vi "Save.vi"(0 "User Manager Model in":refnum<class "User Manager Model.lvclass">, 11 "error in (no error)":errorcluster) -> (4 "User Manager Model out":refnum<class "User Manager Model.lvclass">, 15 "error out":errorcluster)   [LabVIEW 2017, in "User Manager Model.lvlib" / "User Manager Model.lvclass"]
uses:
  User Manager Model.lvclass
  <vilib>/gpm_packages/@cs/persistence/source/XML/XML.lvclass
  C:/Program Files/National Instruments/LabVIEW 2017/vi.lib/gpm_packages/@cs/persistence/source/IPersist/IPersist.lvclass
  User Manager Model.lvclass/User Manager Model.ctl
  Accessors/Read Persistence Path.vi
  <vilib>/gpm_packages/@cs/user-manager/Source/User Configuration Manager Ref/By Ref.lvlib
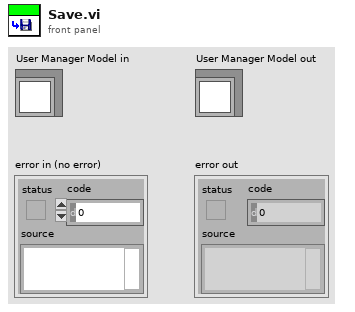
[diagram p1: front panel]
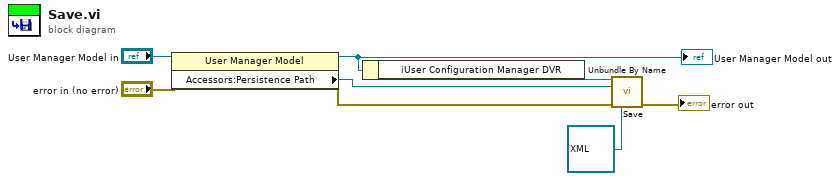
[diagram p0: block diagram]
diagram:
  n1 = property on="Property Node" class="User Manager Model"(reference="User Manager Model in", error in="error in (no error)") -> (reference out=w5:refnum<class "User Manager Model.lvclass">, error out=w2:errorcluster, "Accessors:Persistence Path"=w3:path)
  "User Manager Model out" <- w5
  n2 = Unbundle By Name(w5) -> ("iUser Configuration Manager DVR"=w4:refnum<data-value>)
  n3 = call <vilib>:"Save.vi"("iUser Configuration Manager DVR"=w4, "Path"=w3, "error in"=w2, "Persistence"=refnum<class "XML.lvclass"> refnum ("XML.lvlib:XML.lvclass")) -> ("error out"=→"error out":errorcluster)  [unwired: 10 in, 1 out]
